vi "get Data.vi"(11 "EEPROM in":refnum<class "EEPROM.lvclass">) -> (3 "Data":u8[](array[numeric]))   [LabVIEW 2021, in "EEPROM.lvclass"]
uses:
  EEPROM.lvclass
  EEPROM.lvclass/EEPROM.ctl
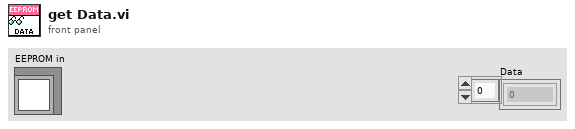
[diagram p1: front panel]
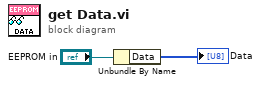
[diagram p0: block diagram]
diagram:
  n1 = Unbundle By Name("EEPROM in") -> ("Data"=→"Data":u8[])
